vi "exnSpectralBlock spectral measurements PSD poly.vi"   [LabVIEW 2020]
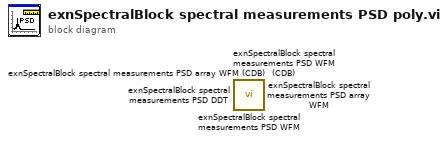
[diagram p0: block diagram]
diagram:
  n1 = call <vilib>:"exnSpectralBlock spectral measurements PSD WFM.vi"() -> ()  [unwired: 13 in, 3 out]
  n2 = call <vilib>:"exnSpectralBlock spectral measurements PSD WFM (CDB).vi"() -> ()  [unwired: 13 in, 3 out]
  n3 = call <vilib>:"exnSpectralBlock spectral measurements PSD DDT.vi"() -> ()  [unwired: 13 in, 3 out]
  n4 = call <vilib>:"exnSpectralBlock spectral measurements PSD array WFM.vi"() -> ()  [unwired: 13 in, 3 out]
  n5 = call <vilib>:"exnSpectralBlock spectral measurements PSD array WFM (CDB).vi"() -> ()  [unwired: 13 in, 3 out]
